vi "Serial_Logic.vi"(8 "error in":errorcluster, 11 "Serial path":path) -> (0 "error out":errorcluster)   [LabVIEW 2017]
panel:
  out "Date":string
  out "String":string
  out "date/time string 2":string
  out "date/time string":string
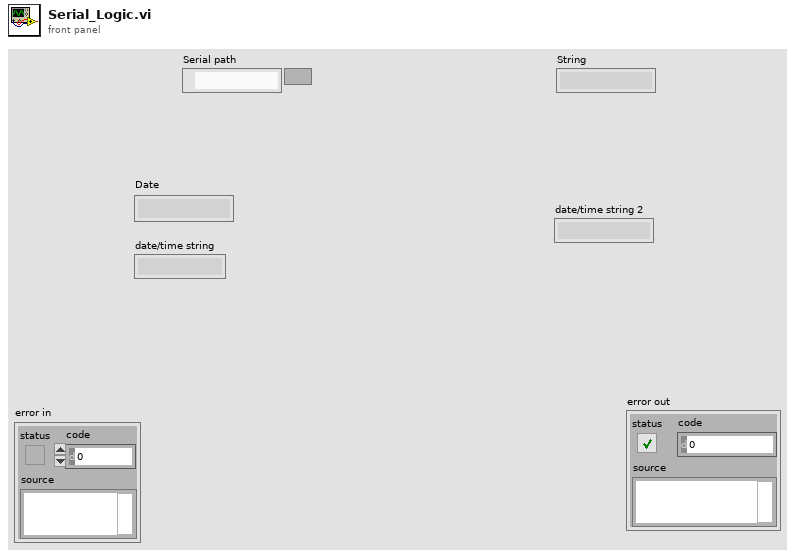
[diagram p1: front panel]
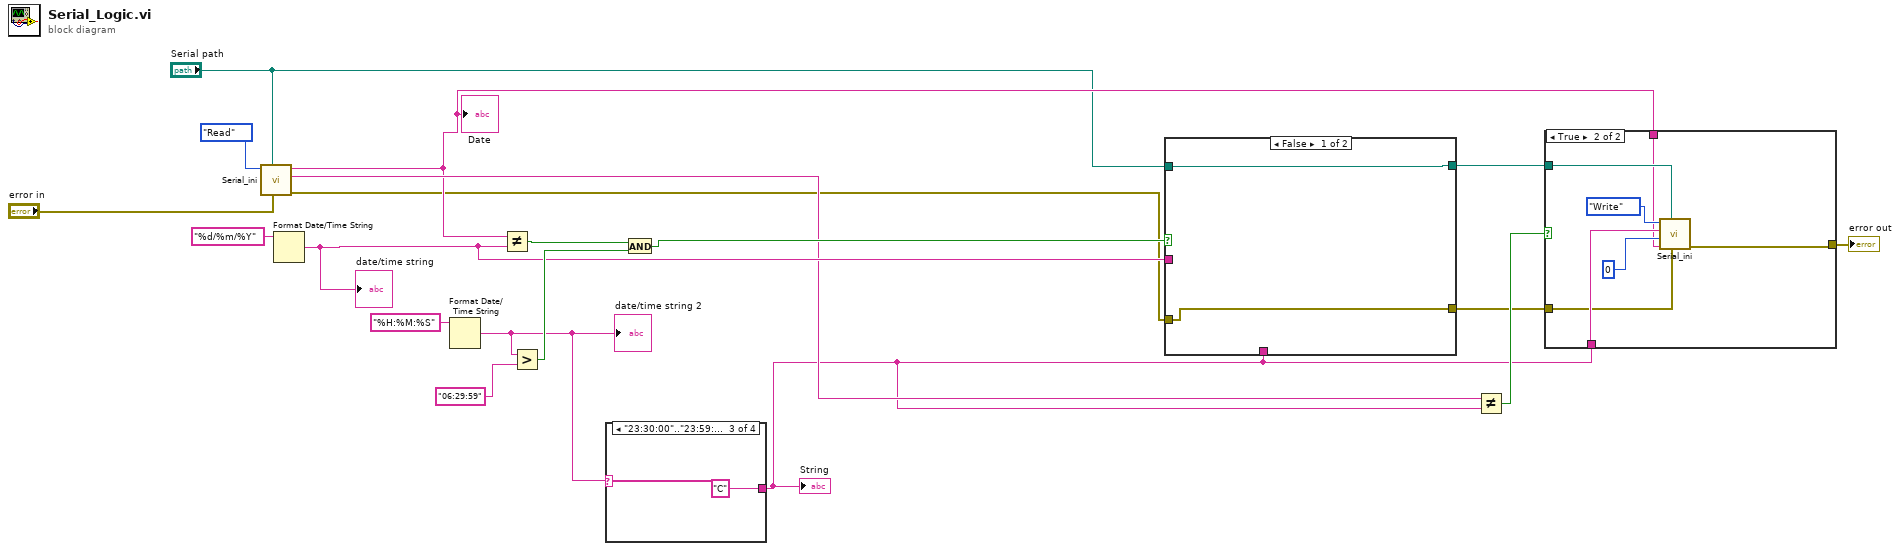
[diagram p0: block diagram]
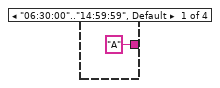
[diagram p3: hidden frame]
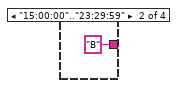
[diagram p4: hidden frame]
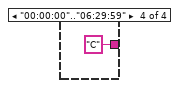
[diagram p5: hidden frame]
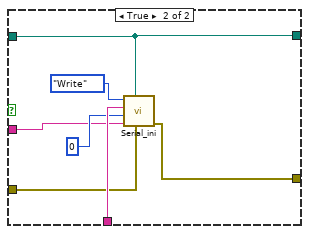
[diagram p6: hidden frame]
diagram:
  n1 = call "Serial_ini.vi"("error in"="error in", "Serial path"="Serial path", "Enum"=enum16{"Write", "Read"}."Read") -> ("error out"=w3:errorcluster, "Shift"=w10:string, "Date"=w6:string)  [unwired: 5 in, 1 out]
  "Date" <- w6
  n2 = Format Date/Time String(time format string (%c)="%d/%m/%Y") -> (date/time string=w11:string)  [unwired: 2 in]
  "date/time string" <- w11
  n3 = Format Date/Time String(time format string (%c)="%H:%M:%S") -> (date/time string=w14:string)  [unwired: 2 in]
  "date/time string 2" <- w14
  n4 = Not Equal?(x=w6, y=w11) -> (x != y?=w13:bool)
  n5 = Greater?(x=w14, y="06:29:59" ("time format string (%c)")) -> (0:w16:bool)
  n6 = case shown="\"23:30:00\"..\"23:59:59\"" w14 {
    tunnel: ["A" "B" "C" "C"] -> w7
    frame "06:30:00".."14:59:59", Default {
    }
    frame "15:00:00".."23:29:59" {
    }
    frame "23:30:00".."23:59:59" {
    }
    frame "00:00:00".."06:29:59" {
    }
  }
  "String" <- w7
  n7 = And(x=w13, y=w16) -> (x .and. y?=w15:bool)
  n8 = case shown="False" w15 {
    tunnel: "Serial path" -> [w25 w28]
    tunnel: w7 -> [_ w31]
    tunnel: w11 -> [_ w29]
    tunnel: [w25 w28] -> w8
    tunnel: [w24 w27] -> w4
    tunnel: w3 -> [w24 w26]
    frame False {
    }
    frame True {
      n9 = call "Serial_ini.vi"("error in"=w26, "Serial path"=w28, "Date"=w29, "Count"=0, "Shift"=w31, "Enum"=enum16{"Write", "Read"}."Write") -> ("error out"=w27:errorcluster)  [unwired: 2 in, 3 out]
    }
  }
  n10 = Not Equal?(x=w10, y=w7) -> (x != y?=w9:bool)
  n11 = case shown="True" w9 {
    tunnel: w8 -> [_ w39]
    tunnel: w7 -> [_ w37]
    tunnel: w6 -> [_ w36]
    tunnel: [w33 w35] -> w1
    tunnel: w4 -> [w33 w34]
    frame False {
    }
    frame True {
      n12 = call "Serial_ini.vi"("error in"=w34, "Serial path"=w39, "Date"=w36, "Count"=0, "Shift"=w37, "Enum"=enum16{"Write", "Read"}."Write") -> ("error out"=w35:errorcluster)  [unwired: 2 in, 3 out]
    }
  }
  "error out" <- w1
